vi "Read Measurement (Quality Power Analysis).vi"(0 "VISA resource name":refnum<visa-resource-name>, 5 "Quality Measurement Type (0: Angle)":i32(ring) items=["Angle", "Apparent", "Crest", "Factor", "Reactive", "Real"], 11 "error in (no error)":errorcluster) -> (4 "VISA resource name out":refnum<visa-resource-name>, 6 "Quality Measurement":dbl, 15 "error out":errorcluster)   [LabVIEW 2015, in "Agilent 2000 3000 X-Series.lvlib"]
doc: "Returns the measurement of a quality power analysis.\n\n<B>Note(s):</B>\nUse <B>Configure Power Analysis (Quality).vi</B> to apply a power analysis."
uses:
  Agilent 2000 3000 X-Series.lvlib
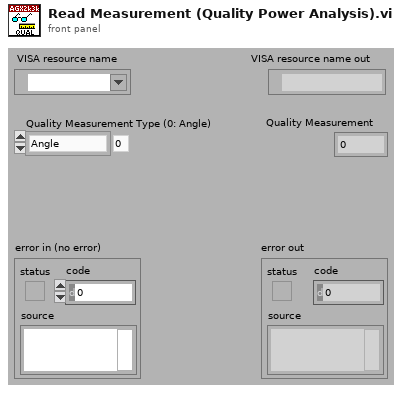
[diagram p1: front panel]
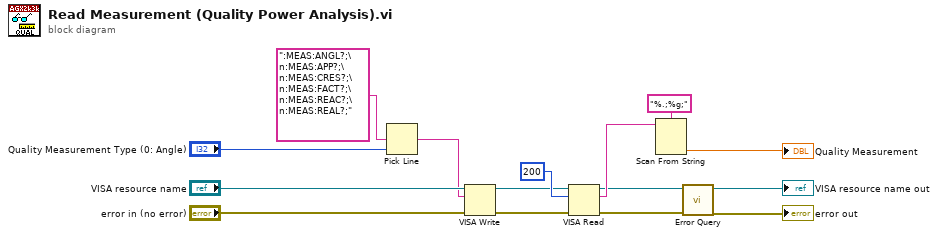
[diagram p0: block diagram]
diagram:
  n1 = Pick Line(multi-line string=":MEAS:ANGL?;\n:MEAS:APP?;\n:MEAS:CRES?;\n:MEAS:FACT?;\n:MEAS:REAC?;\n:MEAS:REAL?;", line index="Quality Measurement Type (0: Angle)") -> (output string=w3:string)  [unwired: 1 out]
  n2 = VISA Write(VISA resource name="VISA resource name", write buffer=w3, error in (no error)="error in (no error)") -> (VISA resource name out=w9:refnum<visa-resource-name>, error out=w8:errorcluster)  [unwired: 1 out]
  n3 = VISA Read(VISA resource name=w9, byte count=u32 200, error in (no error)=w8) -> (VISA resource name out=w6:refnum<visa-resource-name>, read buffer=w10:string, error out=w7:errorcluster)  [unwired: 1 out]
  n4 = Scan From String(format string="%.;%g;", input string=w10) -> (output 1=→"Quality Measurement":dbl)  [unwired: 2 in, 4 out]
  n5 = call "Error Query.vi"("error in (no error)"=w7, "VISA resource name"=w6) -> ("error out"=→"error out":errorcluster, "VISA resource name out"=→"VISA resource name out":refnum<visa-resource-name>)  [unwired: 8 out]
